vi "Drive Controller.vi"(8 "error in":errorcluster) -> ()   [LabVIEW 2019]
doc: "This VI executes continuously carrying out the current operation and responding to updates or new operation requests. It will often contain the timing or control code that is difficult to place directly in TeleOp. This VI generally opens all sensors and motors and isolates the rest of the robot code from knowing implementation details of how the operations are carried out."
uses:
  <vilib>/Rock Robotics/WPI/Framework/Completion Status.ctl
  Drive Setpoints.ctl
  Drive Operations.ctl
  <vilib>/Rock Robotics/WPI/ThirdParty/REV Robotics/SPARK MAX/Typedef/Spark MAX Control Type.ctl
  <vilib>/Rock Robotics/SystemInterfaces/Utilities/FPGA_UtilitiesRead LocalTime.vi
panel:
  in  "Interactive Values":T1
  in  "Buttons":cluster{"Execute Cmd":bool, "Abort Cmd":bool}
  out "Command Timing":cluster{"Start Time (ms)":u32, "Iterations":i32}
  out "Status":T3
  out "Setpoints":T4(graph)
  out "Current\nCmd":string
  # "Tip: The graph shows the motor setpoints. It may also be helpful to observe inputs and sensor values.\nYou may also want to display tuning or debugging controls."
  # "Interactive Command: You may fill in the settings for a command\nand schedule it with the Execute button. You can observe and abort\nany command while fine tuning the code for the controller."
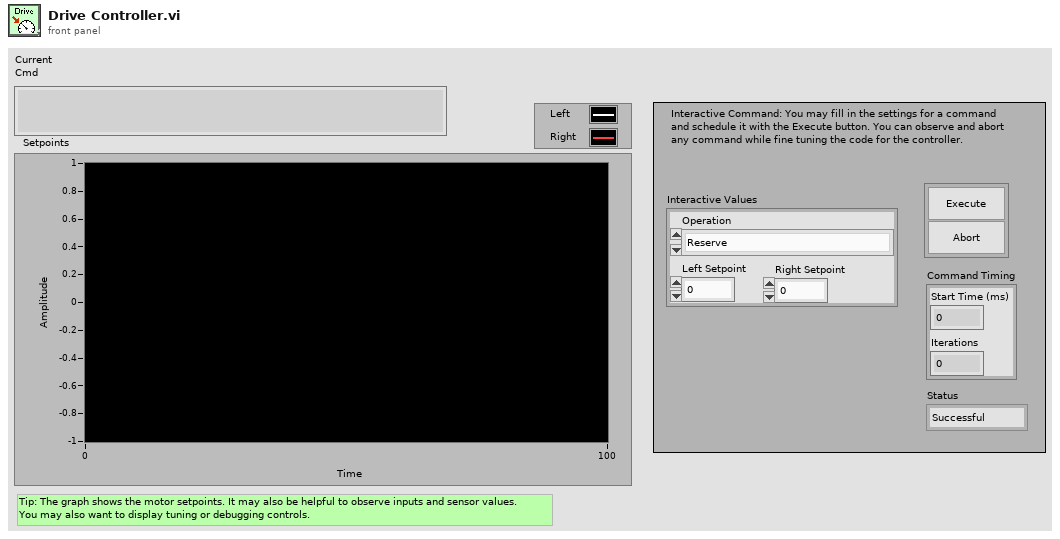
[diagram p1: front panel]
types:
  T1 = typedef "Drive Setpoints.ctl" = cluster{"Operation":T2, "Left Setpoint":dbl, "Right Setpoint":dbl}
  T2 = typedef "Drive Operations.ctl" = enum16{"Reserve", "Read Current", "Immediate", "Play Path"}
  T3 = typedef "Completion Status.ctl" = enum16{"Successful", "Aborted", "Incomplete"}
  T4 = cluster{"Left Setpoint":dbl, "Right Setpoint":dbl}
  T5 = typedef "WPI_MotorControlDeviceRef.ctl" = cluster{"DeviceStatus":errorcluster, "Type":T6, "PWM":cluster{"PWM Channel":T7, "DeadBand":T8}, "CAN":cluster{"Device Number":u8, "SetOutput VI Ref":variant, "GetOutput VI Ref":variant, "Enable VI Ref":variant, "Disable VI Ref":variant, "Data":variant}, "Invert":bool, "DIO PWM":cluster{"PWM \"Enable\" Channel":T7, "DIOChannel":T9, "PWM Rate":dbl}}
  T6 = typedef "WPI_MotorControlType.ctl" = enum16{"PWM", "CAN", "DIO PWM"}
  T7 = typedef "FPGA_DIOPWMChannel.ctl" = enum8{"PWM 0", "PWM 1", "PWM 2", "PWM 3", "PWM 4", "PWM 5", "PWM 6", "PWM 7", "PWM 8", "PWM 9", "PWM MXP 0", "PWM MXP 1", "PWM MXP 2", "PWM MXP 3", "PWM MXP 4", "PWM MXP 5", "PWM MXP 6", "PWM MXP 7", "PWM MXP 8", "PWM MXP 9", "Invalid"}
  T8 = typedef "WPI_PWMDeadband.ctl" = cluster{"Name":string, "maxPositivePwm":i32, "minPositivePwm":i32, "centerPwm":i32, "maxNegativePwm":i32, "minNegativePwm":i32, "angularRange":u16}
  T9 = typedef "FPGA_DIOChannel.ctl" = enum8{"DIO 0", "DIO 1", "DIO 2", "DIO 3", "DIO 4", "DIO 5", "DIO 6", "DIO 7", "DIO 8", "DIO 9", "DIO MXP 0", "DIO MXP 1", "DIO MXP 2", "DIO MXP 3", "DIO MXP 4", "DIO MXP 5", "DIO MXP 6", "DIO MXP 7", "DIO MXP 8", "DIO MXP 9", "DIO MXP 10", "DIO MXP 11", "DIO MXP 12", "DIO MXP 13", "DIO MXP 14", "DIO MXP 15", "SPI Port CS1", "SPI Port CS2", "SPI Port CS3", "SPI Port MISO", "SPI Port MOSI", "Invalid"}
  T10 = typedef "Command Status Info.ctl" = cluster{"Name":string, "Status":T3, "notifier out":T11}
  T11 = typedef "Completion Notifier.ctl" = refnum<notifier>
  T12 = cluster{"SubSystem Data":T1, cluster{"Start Time (ms)":u32, "Iterations":i32}, cluster{"Command Info":T10, "Description":string, "Default Command":T1, "queue out":refnum<queue>, "Subsystem Name":string}}
  T13 = typedef "Spark MAX Control Type.ctl" = enum16{"Percent VBus", "Voltage", "Velocity", "Position", "Smart Motion", "Current", "Smart Velocity"}
  T14 = cluster{"SubSystem Data":T1, cluster{"Start Time (ms)":u32, "Iterations":i32}, "Default Command Arguments":cluster{"Command Info":T10, "Description":string, "Default Command":T1, "queue out":refnum<queue>, "Subsystem Name":string}}
  T15 = cluster{"Don't move motors while reserved":dbl, "Don't move motors while reserved":dbl}
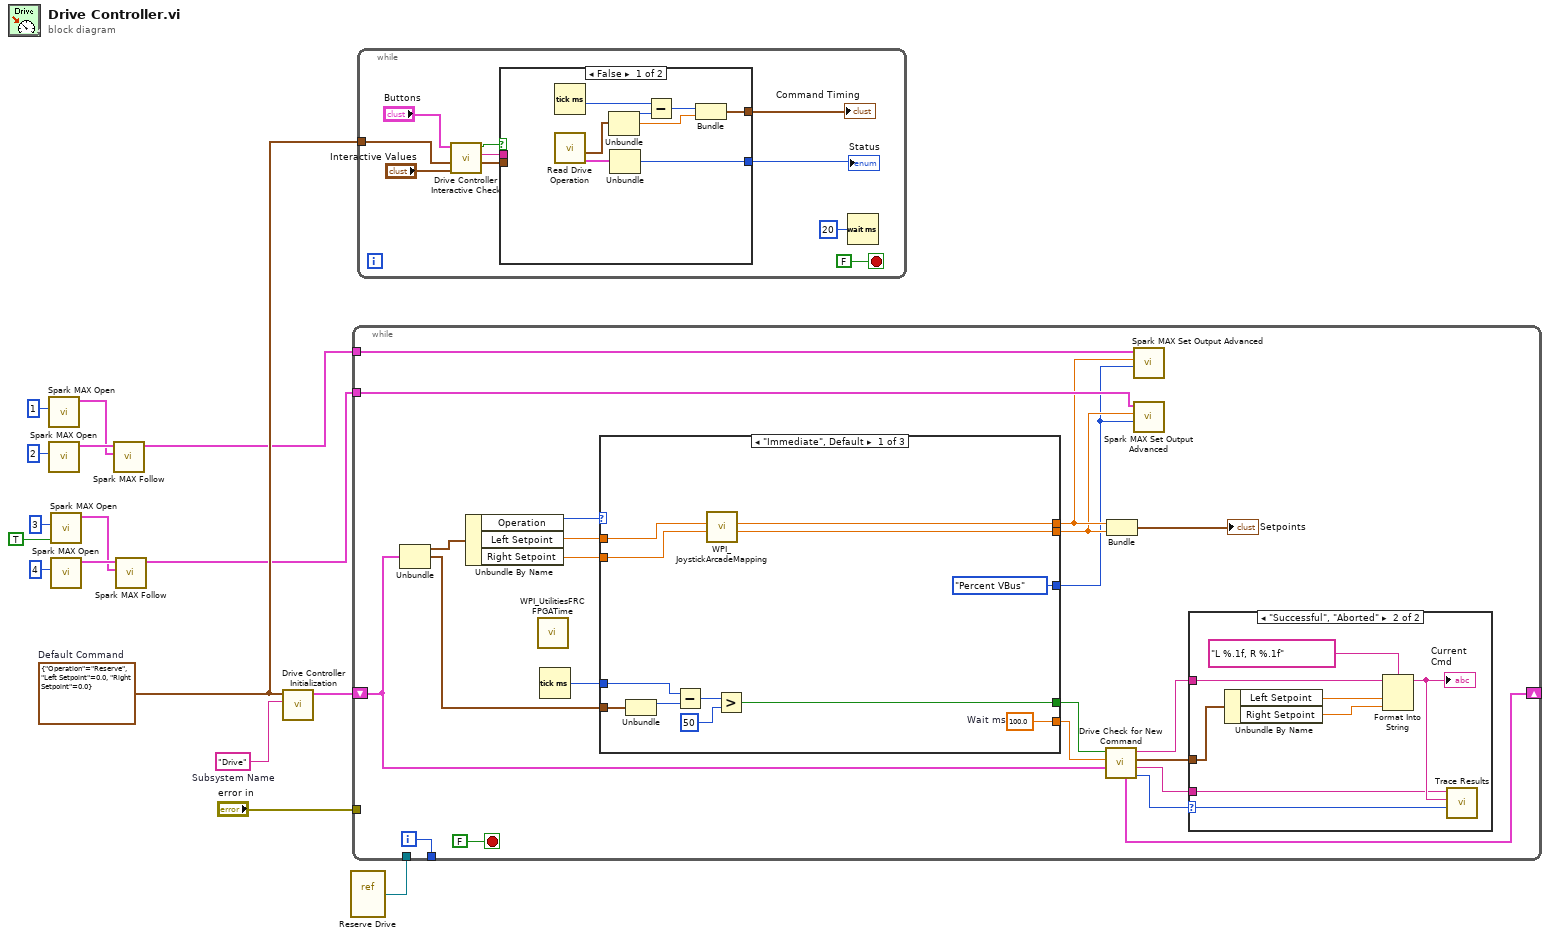
[diagram p0: block diagram]
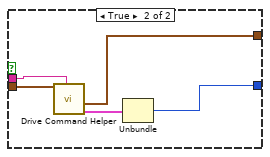
[diagram p2: hidden frame]
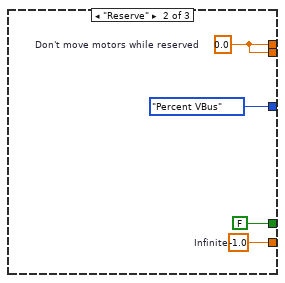
[diagram p4: hidden frame]
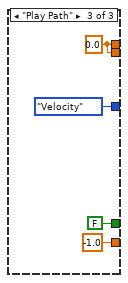
[diagram p5: hidden frame]
diagram:
  w12 = T1 {"Operation"=enum."Reserve", "Left Setpoint"=0.0, "Right Setpoint"=0.0}  # Default Command
  w16 = "Drive"  # Subsystem Name
  n1 = call <vilib>:"Spark MAX Open.vi"("Device Number"=u8 1) -> ("MotorControlDeviceRef"=w8:T5)  [unwired: 9 in, 1 out]
  n2 = call <vilib>:"Spark MAX Open.vi"("Device Number"=u8 2) -> ("MotorControlDeviceRef"=w9:T5)  [unwired: 9 in, 1 out]
  n3 = call <vilib>:"Spark MAX Open.vi"("Invert"=TRUE, "Device Number"=u8 3) -> ("MotorControlDeviceRef"=w4:T5)  [unwired: 8 in, 1 out]
  n4 = call <vilib>:"Spark MAX Open.vi"("Device Number"=u8 4) -> ("MotorControlDeviceRef"=w5:T5)  [unwired: 9 in, 1 out]
  n5 = call <vilib>:"Spark MAX Follow.vi"("Master Controller"=w8, "MotorControlDeviceRef"=w9) -> ("MotorControlDeviceRef"=w2:T5)  [unwired: 8 in, 1 out]
  n6 = call <vilib>:"Spark MAX Follow.vi"("Master Controller"=w4, "MotorControlDeviceRef"=w5) -> ("MotorControlDeviceRef"=w1:T5)  [unwired: 8 in, 1 out]
  n7 = call "Drive Controller Initialization.vi"("Subsystem Name"=w16, "Default Command"=w12) -> ("Current Command"=w14:T12)  [unwired: 9 in]
  n8 = vi-ref "Reserve Drive.vi"() -> (w13:refnum<vi>)
  n9 = while {
    shift-right: [w29] -> _
    shift-left: w14 -> [w22]
    tunnel: [w37] -> _
    tunnel: "error in" -> [_]
    tunnel: w13 -> [_]
    tunnel: w2 -> [w21]
    tunnel: w1 -> [w20]
    i -> [w37]
    stop <- FALSE stop-if-true
    n10 = Unbundle(w22) -> ("SubSystem Data"=w35:T1, w23:cluster{"Start Time (ms)":u32, "Iterations":i32})  [unwired: 1 out]
    n11 = Unbundle By Name(w35) -> ("Operation"=w34:T2, "Left Setpoint"=w33:dbl, "Right Setpoint"=w32:dbl)
    n12 = call <vilib>:"WPI_UtilitiesFRC FPGATime.vi"() -> ()  [unwired: 10 in, 2 out]
    n13 = Tick Count (ms)() -> (millisecond timer value=w31:u32)
    n14 = case shown="\"Immediate\", Default" w34 {
      tunnel: [w58 w62 -1.0 ("Infinite")] -> w28
      tunnel: [w53 FALSE ("ignore previous (F)") FALSE ("ignore previous (F)")] -> w27
      tunnel: w23 -> [w52 _ _]
      tunnel: [w48 w60 w65] -> w19
      tunnel: [w47 w60 w65] -> w18
      tunnel: w33 -> [w50 _ _]
      tunnel: w32 -> [w49 _ _]
      tunnel: w31 -> [w54 _ _]
      tunnel: [Spark_MAX_Control_Type."Percent VBus" ("Control Mode") Spark_MAX_Control_Type."Percent VBus" ("Control Mode") Spark_MAX_Control_Type."Velocity" ("Control Mode")] -> w17
      frame "Immediate", Default {
        w58 = 100.0  # Wait ms
        n15 = Unbundle(w52) -> ("Start Time (ms)"=w55:u32)  [unwired: 1 out]
        n16 = Subtract(x=w54, y=w55) -> (x-y=w56:u32)
        n17 = call <vilib>:"WPI_JoystickArcadeMapping.vi"("Y axis value"=w49, "X axis value"=w50) -> ("Right Motor Value"=w47:dbl, "Left Motor Value"=w48:dbl)  [unwired: 8 in]
        n18 = Greater?(x=w56, y=u8 50 ("Left Motor")) -> (0:w53:bool)
      }
      frame "Reserve" {
        w60 = 0.0  # Don't move motors while reserved
        w62 = -1.0  # Infinite
      }
      frame "Play Path" {
        w65 = 0.0 ("Don't move motors while reserved")
      }
    }
    n19 = call "Drive Check for New Command.vi"("input cluster"=w22, "Wait time (ms)"=w28, "Finished?"=w27) -> ("Completion"=w30:T3, "Subsystem Name"=w24:string, "Current Command"=w25:T1, "Initial Trace String"=w26:string, "Next Command"=w29:T14)  [unwired: 4 in]
    n20 = Bundle("Don't move motors while reserved"=w19, "Don't move motors while reserved"=w18) -> (→"Setpoints":T15)  [unwired: 1 in]
    n21 = call <vilib>:"Spark MAX Set Output Advanced.vi"("Control Mode"=w17, "Setpoint"=w19, "MotorControlDevRef"=w21) -> ()  [unwired: 7 in, 2 out]
    n22 = call <vilib>:"Spark MAX Set Output Advanced.vi"("Control Mode"=w17, "Setpoint"=w18, "MotorControlDevRef"=w20) -> ()  [unwired: 7 in, 2 out]
    n23 = case shown="\"Successful\", \"Aborted\"" w30 {
      selector: w30 -> [_ w46]
      tunnel: w26 -> [_ w41]
      tunnel: w25 -> [_ w42]
      tunnel: w24 -> [_ w39]
      frame "Incomplete", Default {
        # "Continuing current command"
      }
      frame "Successful", "Aborted" {
        # "Report and setup for next command"
        n24 = Unbundle By Name(w42) -> ("Left Setpoint"=w44:dbl, "Right Setpoint"=w45:dbl)
        n25 = Format Into String(format string="L %.1f, R %.1f", initial string=w41, w44, w45) -> (resulting string=w40:string)  [unwired: 1 in, 1 out]
        "Current\nCmd" <- w40
        n26 = call <vilib>:"Trace Results.vi"("Status of previous command"=w46, "Description"=w40, "Subsystem"=w39) -> ()  [unwired: 9 in]
      }
    }
  }
  n27 = while {
    tunnel: w12 -> [w68]
    stop <- FALSE stop-if-true
    n28 = call "Drive Controller Interactive Check.vi"("Interactive Command In"="Interactive Values", "Default Command"=w68, "Buttons"="Buttons") -> ("Interactive Command Out"=w70:T1, "Trace String"=w71:string, "Schedule"=w72:bool)  [unwired: 6 in]
    n29 = case shown="False" w72 {
      tunnel: [w81 w89] -> w73
      tunnel: [w80 w85] -> w74
      tunnel: w71 -> [_ w87]
      tunnel: w70 -> [_ w86]
      frame False {
        n30 = Tick Count (ms)() -> (millisecond timer value=w84:u32)
        n31 = call "Read Drive Operation.vi"() -> ("Command Info"=w78:T10, "SubSystem Data"=w77:T1)  [unwired: 9 in, 1 out]
        n32 = Unbundle(w77) -> ("Operation"=w82:T2, "Left Setpoint"=w79:dbl)  [unwired: 1 out]
        n33 = Unbundle(w78) -> ("Status"=w81:T3)  [unwired: 2 out]
        n34 = Subtract(x=w84, y=w82) -> (x-y=w83:u32)
        n35 = Bundle(w83, "Left Setpoint"=w79) -> (w80:cluster{u32, "Left Setpoint":dbl})  [unwired: 1 in]
      }
      frame True {
        n36 = call "Drive Command Helper.vi"("Description"=w87, "SubSystem Data"=w86) -> ("Command Info Out"=w88:T10, "Command Timing"=w85:cluster{"Start Time (ms)":u32, "Iterations":i32})  [unwired: 7 in, 1 out]
        n37 = Unbundle(w88) -> ("Status"=w89:T3)  [unwired: 2 out]
      }
    }
    "Status" <- w73
    "Command Timing" <- w74
    n38 = Wait (ms)(milliseconds to wait=u32 20) -> ()  [unwired: 1 out]
  }
